vi "TCD to TC.vi"(8 "error in":errorcluster, 10 "Test Configuration":T4(array[cluster]) {"Test Ranking" items=["Low", "Normal", "High"]}, 11 "Test Config Data In":T1[](array[typedef]) {"Test Ranking" items=["Low", "Normal", "High"]}) -> (0 "error out":errorcluster, 3 "Test Config Data Out":T1[](array[typedef]) {"Test Ranking" items=["Low", "Normal", "High"]})   [LabVIEW 2020]
uses:
  <vilib>/addons/analyzer/_analyzerctrls.llb/VIAnCtl Test Config Data.ctl
  <vilib>/addons/analyzer/_analyzerctrls.llb/VIAnCtl TestRanking.ctl
  <vilib>/addons/analyzer/_analyzerctrls.llb/VIAnCtl Config Control Value.ctl
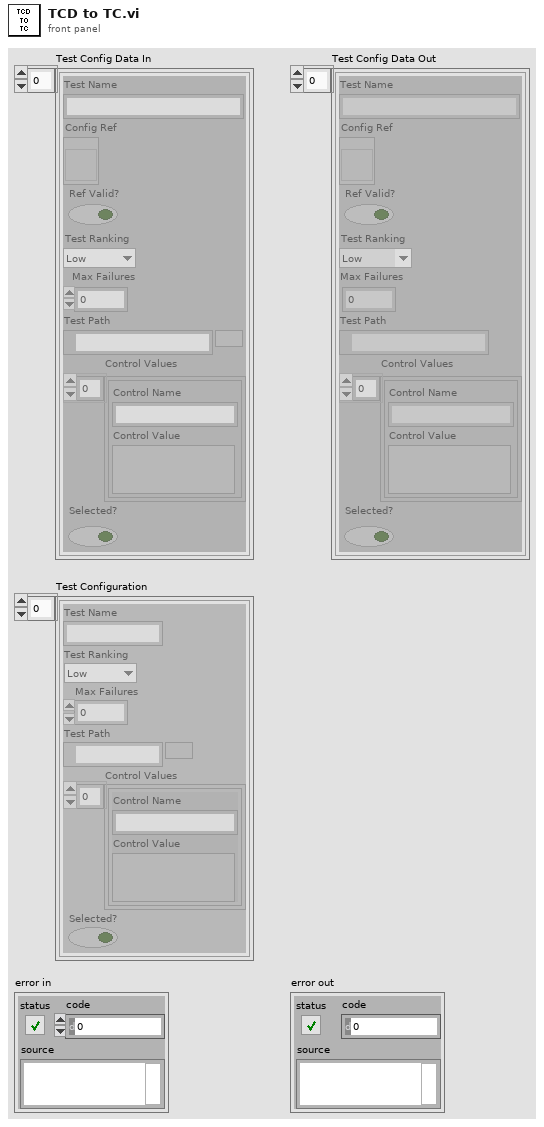
[diagram p1: front panel]
types:
  T1 = typedef "VIAnCtl Test Config Data.ctl" = cluster{"Test Name":string, "Config Ref":refnum<vi>, "Ref Valid?":bool, "Test Ranking":T2, "Max Failures":u32, "Test Path":path, "Control Values":T3[], "Selected?":bool}
  T2 = typedef "VIAnCtl TestRanking.ctl" = u16
  T3 = typedef "VIAnCtl Config Control Value.ctl" = cluster{"Control Name":string, "Control Value":variant}
  T4 = cluster{"Test Name":string, "Test Ranking":T2, "Max Failures":u32, "Test Path":path, "Control Values":T3[], "Selected?":bool}[]
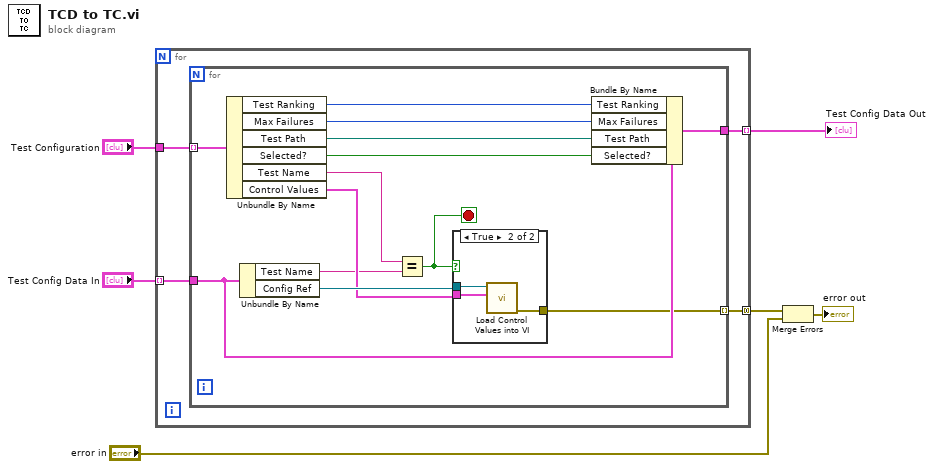
[diagram p0: block diagram]
diagram:
  n1 = for {
    tunnel: "Test Config Data In" -> [w10] mode=indexing
    tunnel: "Test Configuration" -> [w9]
    tunnel: [w8] -> w6 mode=indexing
    tunnel: [w7] -> w3 mode=concatenating
    n2 = for {
      tunnel: w10 -> [w20]
      tunnel: w9 -> [w22] mode=indexing
      tunnel: [w19] -> w8
      tunnel: [w16] -> w7 mode=indexing
      stop <- w15 stop-if-true
      n3 = Unbundle By Name(w22) -> ("Test Ranking"=w14:T2, "Max Failures"=w13:u32, "Test Path"=w12:path, "Selected?"=w11:bool, "Test Name"=w18:string, "Control Values"=w21:T3[])
      n4 = Unbundle By Name(w20) -> ("Test Name"=w17:string, "Config Ref"=w23:refnum<vi>)
      n5 = Equal?(x=w18, y=w17) -> (x = y?=w15:bool)
      n6 = case shown="True" w15 {
        tunnel: w23 -> [_ w26]
        tunnel: w21 -> [_ w25]
        tunnel: [_ w24] -> w16
        frame False {
        }
        frame True {
          n7 = call <vilib>:"Load Control Values into VI.vi"("Control Values"=w25, "VI in"=w26) -> ("error out"=w24:errorcluster)  [unwired: 9 in]
        }
      }
      n8 = Bundle By Name(cluster=w20, "Test Ranking"=w14, "Max Failures"=w13, "Test Path"=w12, "Selected?"=w11) -> (w19:T1)
    }
  }
  "Test Config Data Out" <- w6
  n9 = Merge Errors(w3, "error in") -> (→"error out":errorcluster)
